vi "test_waveform_download.vi"() -> ()   [LabVIEW 2013]
uses:
  _typedefs/daqio-monthly-rollups-JSON.ctl
  _typedefs/daqio-Credentials.ctl
  daqio minimal.lvlib
panel:
  out "error out":errorcluster
  in  "Credentials":T1
  out "value":T2[](array[typedef])
  out "values out":T3(array[cluster])
  in  "End Time":timestamp
  in  "Start Time":timestamp
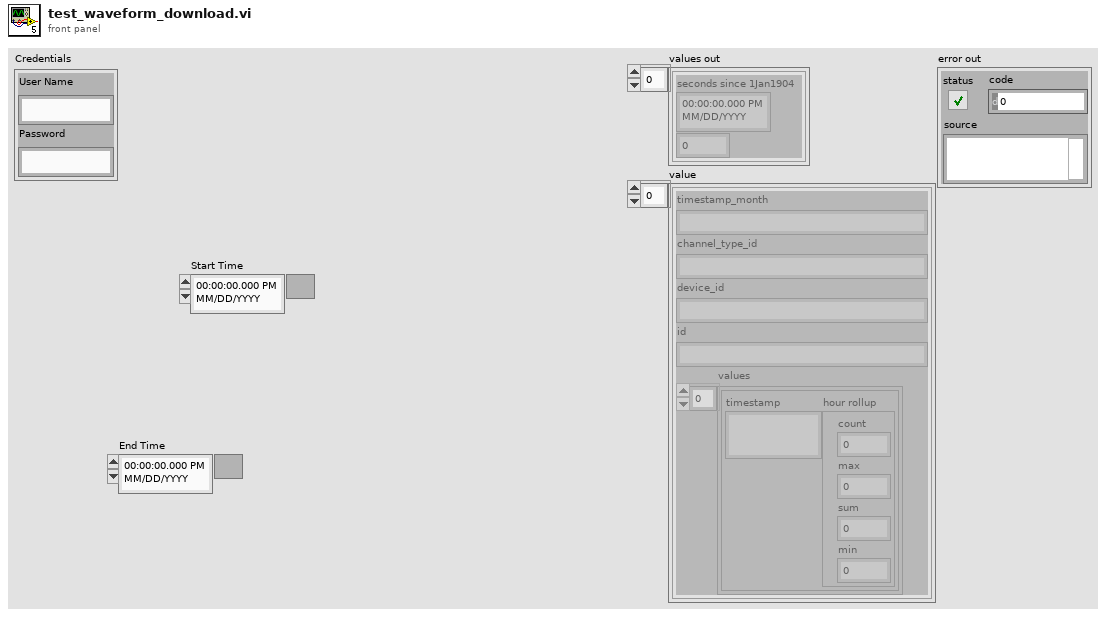
[diagram p1: front panel]
types:
  T1 = typedef "daqio minimal.lvlib/daqio-Credentials.ctl" = cluster{"User Name":string, "Password":string}
  T2 = typedef "daqio minimal.lvlib/daqio-monthly-rollups-JSON.ctl" = cluster{"timestamp_month":string, "channel_type_id":string, "device_id":string, "id":string, "values":cluster{"timestamp":string, "hour rollup":cluster{"count":i32, "max":dbl, "sum":dbl, "min":dbl}}[]}
  T3 = cluster{"seconds since 1Jan1904":timestamp, dbl}[]
  T4 = typedef "daqio minimal.lvlib/daqio-Type.ctl" = cluster{"daq.io ref":T5, "daq.io API Base":string, "Device Type Key":string, "Device Key":string, "Account ID":string, "online":bool}
  T5 = typedef "LabVIEWHTTPClient.lvlib/ClientHandle.ctl" = refnum<k1>
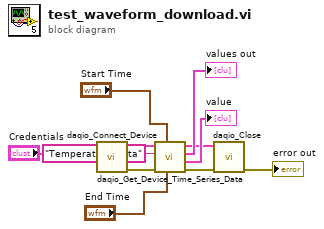
[diagram p0: block diagram]
diagram:
  n1 = call "daqio_Connect_Device.vi"("Credentials"="Credentials") -> ("error out"=w10:errorcluster, "daq.io type out"=w11:T4)  [unwired: 7 in, 2 out]
  n2 = call "daqio_Get_Device_Time_Series_Data.vi"("End Time"="End Time", "Start Time"="Start Time", "error in (no error)"=w10, "Channel ID"="Temperature Data", "daq.io type in"=w11) -> ("error out"=w5:errorcluster, "value"=→"value":T2[], "values out"=→"values out":T3, "daq.io type out"=w4:T4)  [unwired: 3 in]
  n3 = call "daqio_Close.vi"("error in (no error)"=w5, "daq.io type"=w4) -> ("error out"=→"error out":errorcluster)  [unwired: 9 in]
